vi "updateVarto Cluster.vi"(8 "user error in":errorcluster, 9 "variables to update":string[](array[string]), 10 "config array":string[][](array[string]), 11 "Data cluster in":T1) -> (0 "user error out":errorcluster, 3 "Data cluster out":T1)   [LabVIEW 2009]
uses:
  dataCluster.ctl
  <vilib>/vision/Image Controls.llb/IMAQ Image.ctl
  DataQueueTypeDef.ctl
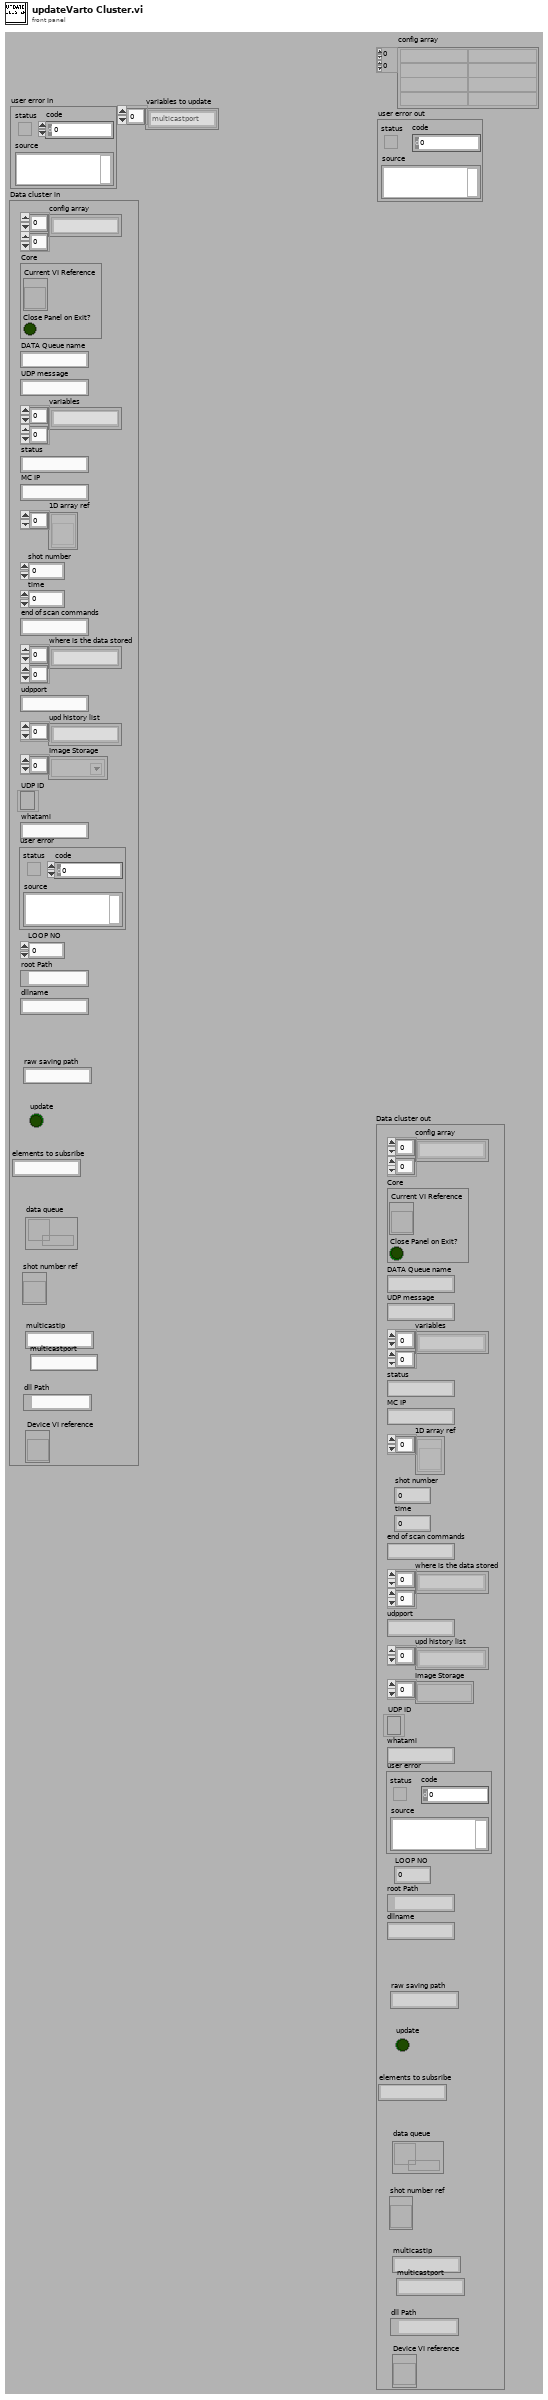
[diagram p1: front panel]
types:
  T1 = typedef "dataCluster.ctl" = cluster{"config array":string[][], "Core":cluster{"Current VI Reference":refnum<vi>, "Close Panel on Exit?":bool}, "DATA Queue name":string, "UDP message":string, "variables":string[][], "status":string, "MC IP":string, "1D array ref":refnum<vi>[], "shot number":i32, "time":u32, "end of scan commands":string, "where is the data stored":string[][], "udpport":string, "upd history list":string[], "Image Storage":T2[], "UDP ID":refnum<k16>, "whatami":string, "user error":errorcluster, "LOOP NO":u32, "root Path":path, "dllname":string, "raw saving path":string, "update":bool, "elements to subsribe":string, "data queue":refnum<queue>, "shot number ref":refnum<vi>, "multicastip":string, "multicastport":string, "dll Path":path, "Device VI reference":refnum<vi>}
  T2 = typedef "IMAQ Image.ctl" = refnum<image>
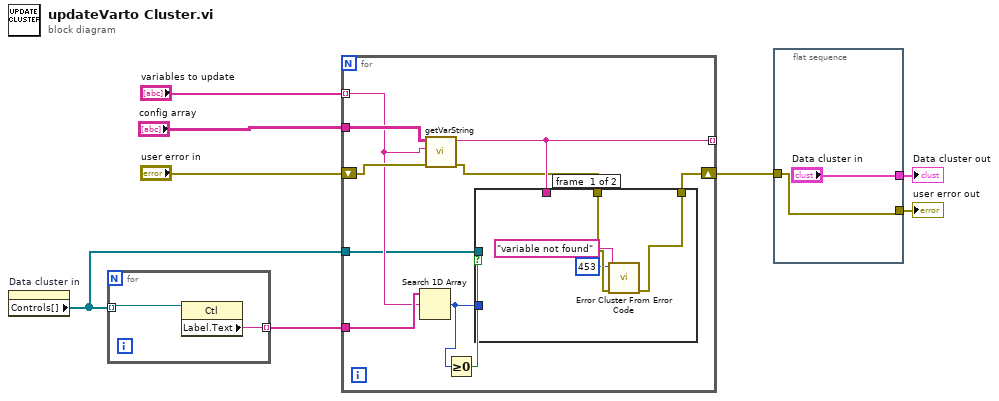
[diagram p0: block diagram]
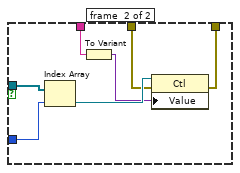
[diagram p2: hidden frame]
diagram:
  n1 = property on="Data cluster in" class="Clust (strict)"() -> ("Controls[]"=w5:refnum<vi>[])  [unwired: 2 in, 2 out]
  n2 = for {
    tunnel: w5 -> [w10] mode=indexing
    tunnel: [w9] -> w6 mode=indexing
    n3 = property class="Ctl"(reference=w10) -> ("Label.Text"=w9:string)  [unwired: 1 in, 2 out]
  }
  n4 = for {
    tunnel: "config array" -> [w20]
    tunnel: "variables to update" -> [w17] mode=indexing
    shift-right: [w13] -> w3
    shift-left: "user error in" -> [w19]
    tunnel: [w15] -> _ mode=indexing
    tunnel: w6 -> [w18]
    tunnel: w5 -> [w16]
    n5 = Search 1D Array(1D array=w18, element=w17) -> (index of element=w12:i32)  [unwired: 1 in]
    n6 = call "getVarString.vi"("user error in"=w19, "element"=w17, "settings"=w20) -> ("user error out"=w14:errorcluster, "value"=w15:string)  [unwired: 3 in]
    n7 = Greater Or Equal To 0?(x=w12) -> (x >= 0?=w11:bool)
    n8 = case shown="False" w11 {
      tunnel: w16 -> [_ w31]
      tunnel: w12 -> [_ w30]
      tunnel: w15 -> [_ w28]
      tunnel: w14 -> [w24 w26]
      tunnel: [w23 w25] -> w13
      frame #0 {
        n9 = call <vilib>:"Error Cluster From Error Code.vi"("error in (no error)"=w24, "error message (\"\")"="variable not found" ("error message (\"\")"), "error code (0)"=453) -> ("error out"=w23:errorcluster)  [unwired: 6 in]
      }
      frame #1 {
        n10 = Index Array(array=w31, index=w30) -> (element=w29:refnum<vi>)
        n11 = To Variant(anything=w28) -> (Variant=w27:variant)
        n12 = property class="Ctl"(reference=w29, error in=w26, "Value"=w27) -> (error out=w25:errorcluster)  [unwired: 1 out]
      }
    }
  }
  n13 = flat-sequence {
    tunnel: w3 -> [w32]
    tunnel: ["Data cluster in"] -> w2
    tunnel: [w32] -> w1
    frame #0 {
    }
  }
  "Data cluster out" <- w2
  "user error out" <- w1
